vi "Example Authenticate.vi"() -> ()   [LabVIEW 2010]
uses:
  C:/tf/play/labview/Tinkerforge.dll
panel:
  out "connection events":string[](array[string])
  in  "secret":string="My Authentication Secret!"
  out "enumeration events":string[](array[string])
  in  "stop":bool
  in  "port":i32=4223
  in  "host":string="localhost"
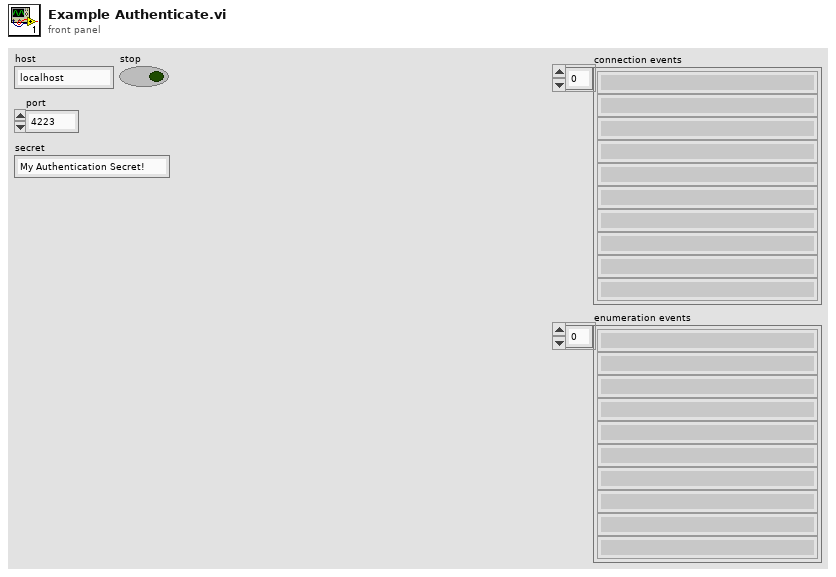
[diagram p1: front panel]
types:
  T1 = cluster{"uid":string, "connectedUid":string, "position":u16, "hardwareVersion":i16[], "firmwareVersion":i16[], "deviceIdentifier":i32, "enumerationType":i16}
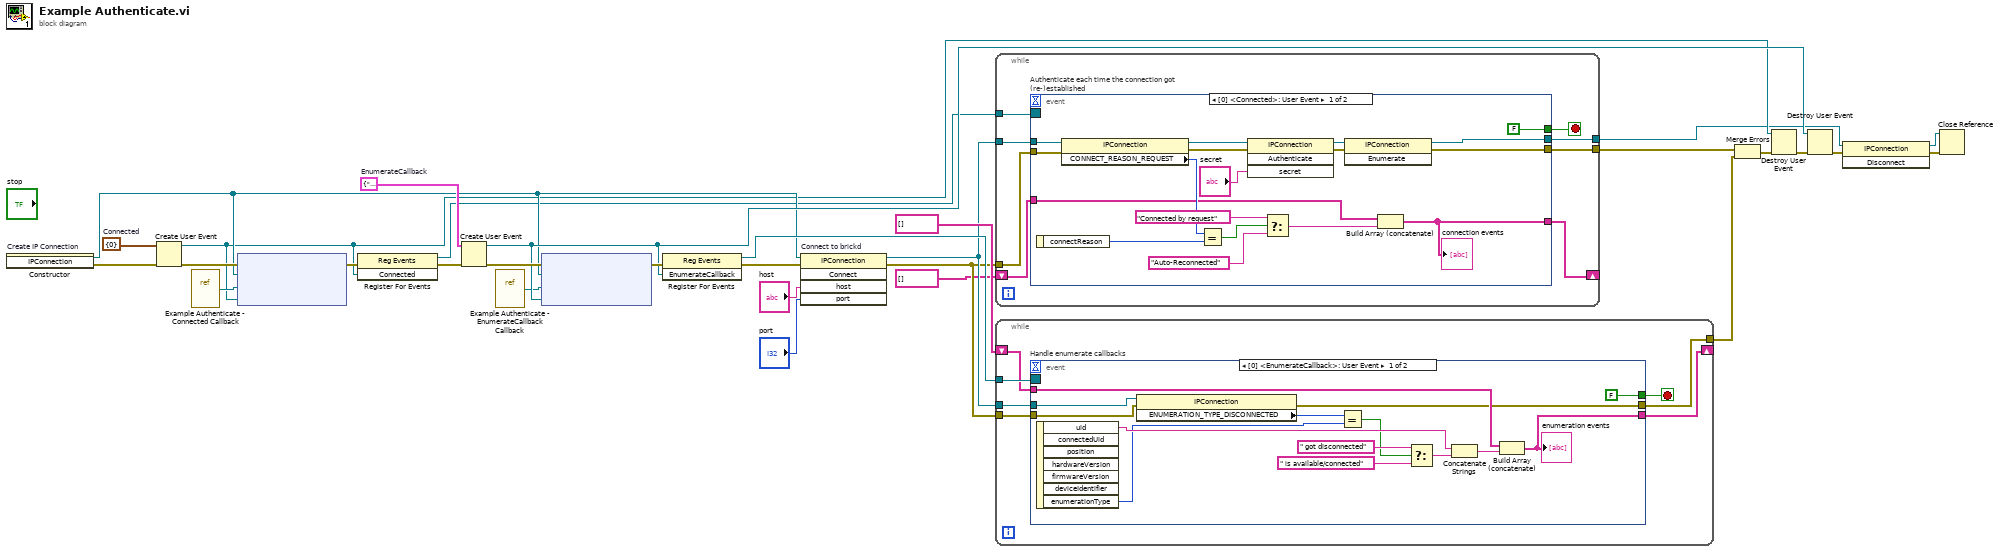
[diagram p0: block diagram]
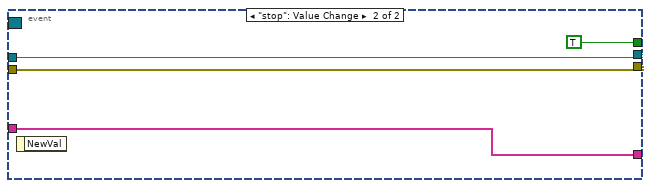
[diagram p2: hidden frame]
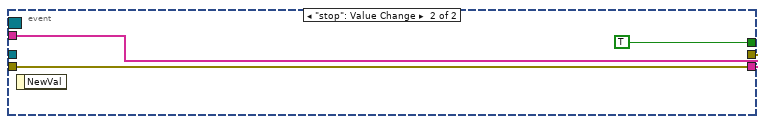
[diagram p3: hidden frame]
diagram:
  w17 = cluster{"connectReason":i16} {"connectReason"=0}  # Connected
  w22 = T1 {"uid"="", "connectedUid"="", "position"=0, "hardwareVersion"=[], "firmwareVersion"=[], "deviceIdentifier"=0, "enumerationType"=0}  # EnumerateCallback
  n1 = constructor on="Create IP Connection" class="IPConnection"() -> (reference out=w12:refnum<k24>, error out=w16:errorcluster)  [unwired: 3 in, 1 out]
  n2 = Create User Event(user event datatype=w17, error in=w16) -> (user event=w8:refnum<user-event>, error out=w18:errorcluster)
  n3 = vi-ref "Example Authenticate - Connected Callback.vi"() -> ("vi reference"=w15:refnum<vi>)
  n4 = node ("Register Event Callback")(w18, w12, w15, w8) -> (w14:errorcluster)  [unwired: 1 in, 1 out]
  n5 = register-events(error in=w14, w8) -> (reference out=w10:refnum<event-registration>, error out=w13:errorcluster)  [unwired: 1 in]
  n6 = Create User Event(user event datatype=w22, error in=w13) -> (user event=w23:refnum<user-event>, error out=w26:errorcluster)
  n7 = vi-ref "Example Authenticate - EnumerateCallback Callback.vi"() -> ("vi reference"=w19:refnum<vi>)
  n8 = node ("Register Event Callback")(w26, w12, w19, w23) -> (w25:errorcluster)  [unwired: 1 in, 1 out]
  n9 = register-events(error in=w25, w23) -> (reference out=w24:refnum<event-registration>, error out=w11:errorcluster)  [unwired: 1 in]
  n10 = invoke on="Connect to brickd" class="IPConnection" method="Connect"(reference=w12, error in=w11, "host"="host", "port"="port") -> (reference out=w7:refnum<k24>, error out=w6:errorcluster)  [unwired: 1 in, 3 out]
  n11 = while {
    tunnel: w10 -> [w38]
    tunnel: w7 -> [w36]
    tunnel: w6 -> [w35]
    tunnel: [w34] -> w5
    tunnel: [w33] -> w4
    shift-right: [w31] -> _
    shift-left: string[] [] -> [w32]
    stop <- w37 stop-if-true
    n12 = event "Authenticate each time the connection got (re-)established" shown="[0] <Connected>: User Event" {
      selector: w38 -> [_ _]
      dyn-events: _ -> [_ _]
      timeout: _ -> [_ _]
      tunnel: [FALSE TRUE] -> w37
      tunnel: w36 -> [w54 w59]
      tunnel: w35 -> [w53 w58]
      tunnel: [w39 w59] -> w34
      tunnel: [w41 w58] -> w33
      tunnel: w32 -> [w45 w57]
      tunnel: [w40 w57] -> w31
      event User Event {
        n13 = event-data() -> ("connectReason"=w49:i16)  [unwired: 1 in]
        n14 = property class="IPConnection"(reference=w54, error in=w53) -> (reference out=w51:refnum<k24>, error out=w52:errorcluster, "CONNECT_REASON_REQUEST"=w50:i16)
        n15 = Equal?(x=w50, y=w49) -> (x = y?=w48:bool)
        n16 = invoke class="IPConnection" method="Authenticate"(reference=w51, error in=w52, "secret"="secret") -> (reference out=w42:refnum<k24>, error out=w43:errorcluster)  [unwired: 1 in, 2 out]
        n17 = Select(t="Connected by request", s=w48, f="Auto-Reconnected") -> (s? t:f=w44:string)
        n18 = invoke class="IPConnection" method="Enumerate"(reference=w42, error in=w43) -> (reference out=w39:refnum<k24>, error out=w41:errorcluster)  [unwired: 1 in, 1 out]
        n19 = Build Array (concatenate)(w45, w44) -> (w40:string[])
        "connection events" <- w40
      }
      event "stop": Value Change {
        n20 = event-data() -> ()  [unwired: 1 in, 1 out]
      }
    }
  }
  n21 = while {
    tunnel: w24 -> [w67]
    tunnel: [w66] -> w2
    tunnel: w6 -> [w65]
    shift-right: [w62] -> _
    shift-left: string[] [] -> [w63]
    tunnel: w7 -> [w61]
    stop <- w64 stop-if-true
    n22 = event "Handle enumerate callbacks" shown="[0] <EnumerateCallback>: User Event" {
      selector: w67 -> [_ _]
      dyn-events: _ -> [_ _]
      timeout: _ -> [_ _]
      tunnel: [w72 w82] -> w66
      tunnel: w65 -> [w73 w82]
      tunnel: [FALSE TRUE] -> w64
      tunnel: w63 -> [w77 w83]
      tunnel: [w76 w83] -> w62
      tunnel: w61 -> [w74 _]
      event User Event {
        n23 = event-data() -> ("uid"=w80:string, "enumerationType"=w69:i16)  [unwired: 1 in, 5 out]
        n24 = property class="IPConnection"(reference=w74, error in=w73) -> (error out=w72:errorcluster, "ENUMERATION_TYPE_DISCONNECTED"=w68:i16)  [unwired: 1 out]
        n25 = Equal?(x=w68, y=w69) -> (x = y?=w70:bool)
        n26 = Select(t=" got disconnected", s=w70, f=" is available/connected") -> (s? t:f=w75:string)
        n27 = Concatenate Strings(w80, w75) -> (w71:string)
        n28 = Build Array (concatenate)(w77, w71) -> (w76:string[])
        "enumeration events" <- w76
      }
      event "stop": Value Change {
        n29 = event-data() -> ()  [unwired: 1 in, 1 out]
      }
    }
  }
  n30 = Merge Errors(w4, w2) -> (w3:errorcluster)
  n31 = Destroy User Event(user event=w8, error in=w3) -> (error out=w9:errorcluster)
  n32 = Destroy User Event(user event=w23, error in=w9) -> (error out=w21:errorcluster)
  n33 = invoke class="IPConnection" method="Disconnect"(reference=w5, error in=w21) -> (reference out=w27:refnum<k24>, error out=w28:errorcluster)  [unwired: 1 in, 1 out]
  n34 = Close Reference(reference=w27, error in (no error)=w28) -> ()  [unwired: 1 out]
